vi "ESP301_Close.vi"(8 "entrée d'erreur (pas d'erreur)":errorcluster, 11 "référence":refnum<k24>) -> (0 "sortie d'erreur":errorcluster)   [LabVIEW 2019]
uses:
  Newport.ESP301.CommandInterface
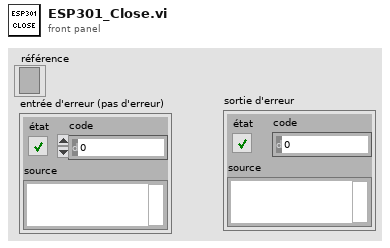
[diagram p1: front panel]
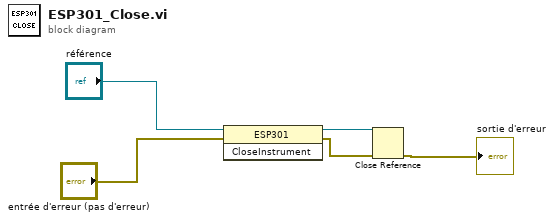
[diagram p0: block diagram]
diagram:
  n1 = invoke on="Nœud de méthode" class="ESP301" method="CloseInstrument"(reference="référence", error in="entrée d'erreur (pas d'erreur)") -> (reference out=w3:refnum<k24>, error out=w2:errorcluster)  [unwired: 1 in, 1 out]
  n2 = Close Reference(reference=w3, error in (no error)=w2) -> (error out=→"sortie d'erreur":errorcluster)
